vi "Shutdown HW.vi"(8 "error in (no error)":errorcluster, 11 "USB Camera in":refnum<class "USB Camera.lvclass">) -> (0 "error out":errorcluster, 3 "USB Camera out":refnum<class "USB Camera.lvclass">)   [LabVIEW 2020, in "USB Camera.lvclass"]
uses:
  USB Camera.lvclass
  USB Camera.lvclass/USB Camera.ctl
  Camera.lvclass
  <vilib>/vision/driver/NI_Vision_Acquisition_Software.lvlib
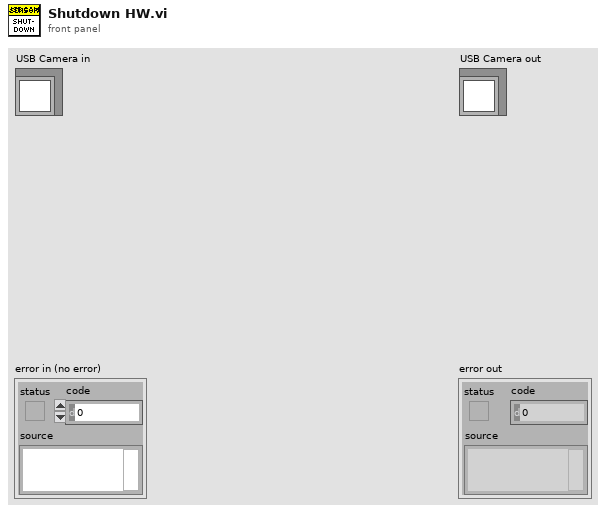
[diagram p1: front panel]
types:
  T1 = typedef "IMAQdx.ctl" = refnum<k21>
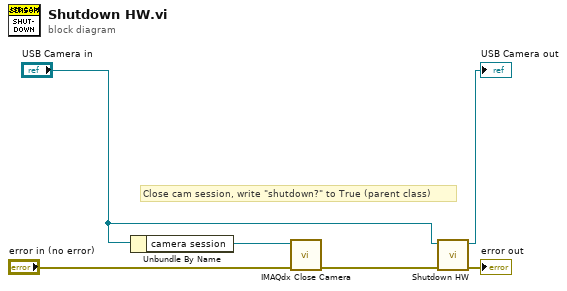
[diagram p0: block diagram]
diagram:
  # "Close cam session, write \"shutdown?\" to True (parent class)"
  n1 = Unbundle By Name("USB Camera in") -> ("camera session"=w2:T1)
  n2 = call <vilib>:"IMAQdx Close Camera.vi"("error in"="error in (no error)", "Session In"=w2) -> ("error out"=w3:errorcluster)  [unwired: 9 in]
  n3 = call-parent "Shutdown HW.vi"("error in (no error)"=w3, "Camera in"="USB Camera in") -> ("error out"=→"error out":errorcluster, "Camera out"=→"USB Camera out":refnum<class "USB Camera.lvclass">)  [unwired: 8 in]
